vi "Test.vi"() -> ()   [LabVIEW 2021]
panel:
  out "element 3":dbl
  out "element 2":dbl
  out "element":dbl
  in  "stop":bool
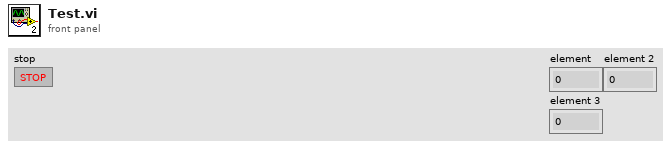
[diagram p1: front panel]
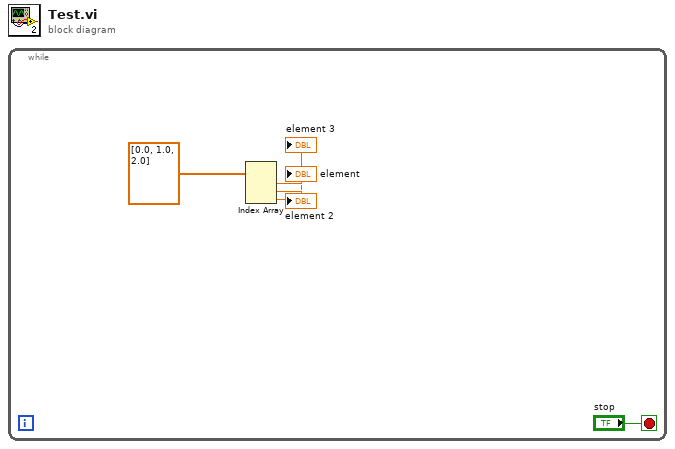
[diagram p0: block diagram]
diagram:
  n1 = while {
    stop <- "stop" stop-if-true
    n2 = Index Array(array=dbl[] [0.0, 1.0, 2.0]) -> (element #1=→"element":dbl, element #2=→"element 2":dbl, element #3=→"element 3":dbl)  [unwired: 3 in]
  }
